vi "m1m3_flushSamplesEvent_HardpointMonitorState.vi"(8 "error in (no error)":errorcluster) -> (0 "error out":errorcluster, 3 "function return":i32)   [LabVIEW 2016, in "SALLV_m1m3.lvlib"]
doc: "int m1m3_shm_flushSamplesEvent_HardpointMonitorStateLV();"
uses:
  SALLV_m1m3.lvlib
  SALLV_m1m3.so
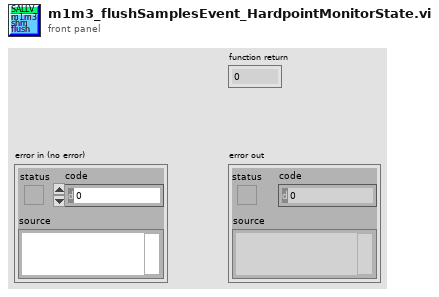
[diagram p1: front panel]
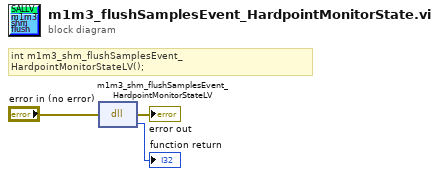
[diagram p0: block diagram]
diagram:
  # "int m1m3_shm_flushSamplesEvent_HardpointMonitorStateLV();"
  n1 = dll-call lib="opt/CODE/SALLV_m1m3/SALLV_m1m3.*" fn="m1m3_shm_flushSamplesEvent_HardpointMonitorStateLV"(error in="error in (no error)") -> (error out=→"error out":errorcluster, →"function return":i32)  [unwired: 2 in, 1 out]
